vi "Read Resource Data ref.vi"(8 "error in (no error)":errorcluster, 11 "VI Data in":refnum<class "VI Data.lvclass">) -> (0 "error out":errorcluster, 2 "Resource Data ref":refnum<data-value>, 3 "VI Data out":refnum<class "VI Data.lvclass">)   [LabVIEW 2013, in "SET Project Data.lvlib" / "VI Data.lvclass"]
uses:
  VI Data.lvclass
  Resource Data Class/Resource Data.lvclass
  VI Data.lvclass/VI Data.ctl
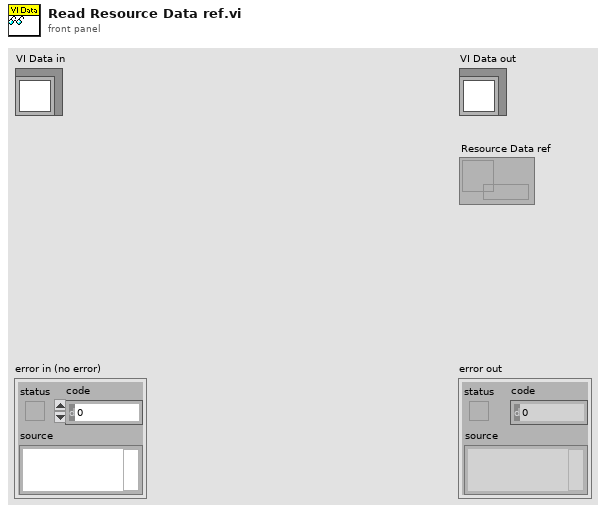
[diagram p1: front panel]
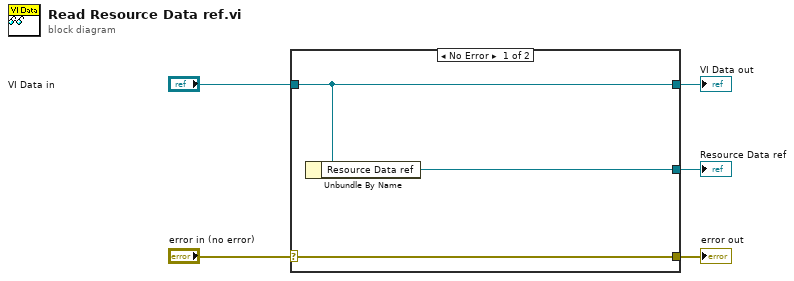
[diagram p0: block diagram]
diagram:
  n1 = case shown="No Error" "error in (no error)" {
    selector: "error in (no error)" -> [w8 w9]
    tunnel: [w8 w9] -> w4
    tunnel: [w7 w10] -> w2
    tunnel: "VI Data in" -> [w7 w10]
    tunnel: [w6 _] -> w1
    frame No Error {
      n2 = Unbundle By Name(w7) -> ("Resource Data ref"=w6:refnum<data-value>)
    }
    frame Error {
    }
  }
  "error out" <- w4
  "VI Data out" <- w2
  "Resource Data ref" <- w1
